vi "WPI_DashboardUpdate Table Values.vi"(11 "Data Values":T5(array[cluster])) -> ()   [LabVIEW 2017]
uses:
  <vilib>/Rock Robotics/Network Tables/Protocol Operations.ctl
  <vilib>/Rock Robotics/Network Tables/Field Data.ctl
  <vilib>/Rock Robotics/Network Tables/Field Type.ctl
  <vilib>/Rock Robotics/Network Tables/Sequence.ctl
  <vilib>/Rock Robotics/WPI/Dashboard/WPI_DashboardLogging Global.vi
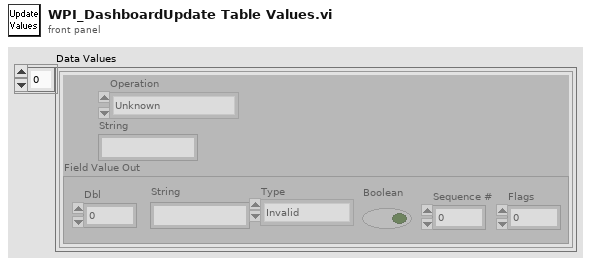
[diagram p1: front panel]
types:
  T1 = typedef "Protocol Operations.ctl" = enum16{"Unknown", "Keep Alive", "Client Hello", "Version not supported", "Server Hello Complete", "Assign", "Update", "No Op", "Server Hello", "Client Hello Complete", "Update Flags", "Delete Entry", "Delete All", "RPC Exec", "RPC Response"}
  T2 = typedef "Field Data.ctl" = cluster{"Dbl":dbl, "String":string, "Type":T3, "Boolean":bool, "Sequence #":T4, "Flags":u8}
  T3 = typedef "Field Type.ctl" = enum8{"Invalid", "Bool", "Numeric", "String", "Raw", "Boolean Array", "Numeric Array", "String Array", "RPC"}
  T4 = typedef "Sequence.ctl" = u16
  T5 = cluster{"Operation":T1, "String":string, "Field Value Out":T2}[]
  T6 = cluster{"Operation":T1, "String":string, "Field Value Out":T2}
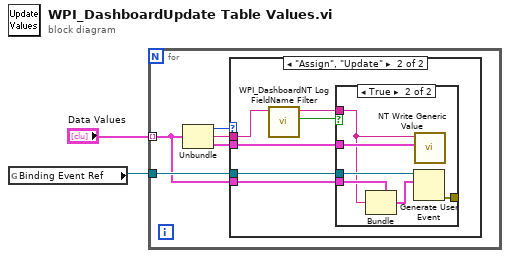
[diagram p0: block diagram]
diagram:
  n1 = global read "WPI_DashboardLogging Global.vi" "Binding Event Ref"() -> (w1:refnum<user-event>)
  n2 = for {
    tunnel: "Data Values" -> [w3] mode=indexing
    tunnel: w1 -> [w4]
    n3 = Unbundle(w3) -> ("Operation"=w7:T1, "String"=w6:string, "Field Value Out"=w5:T2)
    n4 = case shown="\"Assign\", \"Update\"" w7 {
      tunnel: w6 -> [_ w13]
      tunnel: w5 -> [_ w12]
      tunnel: w4 -> [_ w10]
      tunnel: w3 -> [_ w11]
      frame Default {
      }
      frame "Assign", "Update" {
        n5 = call <vilib>:"WPI_DashboardNT Log FieldName Filter.vi"("Name in"=w13) -> ("Success"=w8:bool, "Name out"=w9:string)  [unwired: 9 in]
        n6 = case shown="True" w8 {
          tunnel: w12 -> [_ w19]
          tunnel: w11 -> [_ w17]
          tunnel: w10 -> [_ w18]
          tunnel: w9 -> [_ w15]
          tunnel: [_ w14] -> _
          frame False {
            # "bogus\ncache\nindex"
          }
          frame True {
            n7 = Bundle(cluster=w17, "String"=w15) -> (w16:T6)  [unwired: 2 in]
            n8 = Generate User Event(user event=w18, event data cluster=w16) -> (error out=w14:errorcluster)  [unwired: 2 in, 1 out]
            n9 = call <vilib>:"NT Write Generic Value.vi"("Field Value"=w19, "Name"=w15) -> ()  [unwired: 9 in, 1 out]
          }
        }
      }
    }
  }
